vi "CRYGet Resolution_Steps of Curves.vi"(11 "Curve In":T1={"Name"="", "Curve"=[], "X data"=1, "Y data"=1, "Z data"=1, "X axis"=0, "Y axis"=1, "Z axis"=1, "X unit"="Hz", "Y unit"="", "Z unit"="deg.", "X dB ref"=1.0, "Y dB ref"=1.0, "Z dB ref"=1.0, "single val"=FALSE, "protected"=FALSE, "display X"=TRUE, "display Y"=TRUE, "display Z"=TRUE, "Test Info"="", "Step No."=0, "Plot Settings"={"Color"=0, "Interpolation"=0, "Point Style"=0, "Line Style"=0, "Point Color"=0, "Line Width"=0, "Bar Plot Style"=0, "Fill To"=0}, "AutoProtect"=FALSE} {"Z data" items=["dB", "Lin"]; "X data" items=["dB", "Lin"]; "Y data" items=["dB", "Lin"]; "Z dB ref" format="%.1f"; "Z axis" items=["Log", "Lin"]; "X dB ref" format="%.1f"; "X axis" items=["Log", "Lin"]; "Y axis" items=["Log", "Lin"]; "Y dB ref" format="%.1f"; "Curve"."z" format="%.2f"; "Curve"."y" format="%.2f"; "Curve"."x" format="%.2f"}) -> (1 "Steps Out":i32, 3 "Original Resolution Out":string)   [LabVIEW 2013]
uses:
  Typedef Control/CRYData Cluster.ctl
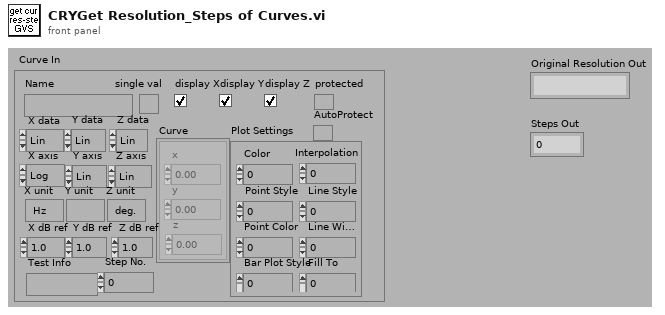
[diagram p1: front panel]
types:
  T1 = typedef "CRYData Cluster.ctl" = cluster{"Name":string, "Curve":cluster{"x":dbl, "y":dbl, "z":dbl}[], "X data":u16, "Y data":u16, "Z data":u16, "X axis":u16, "Y axis":u16, "Z axis":u16, "X unit":string, "Y unit":string, "Z unit":string, "X dB ref":dbl, "Y dB ref":dbl, "Z dB ref":dbl, "single val":bool, "protected":bool, "display X":bool, "display Y":bool, "display Z":bool, "Test Info":string, "Step No.":i32, "Plot Settings":cluster{"Color":u32, "Interpolation":u8, "Point Style":u8, "Line Style":u8, "Point Color":u32, "Line Width":u8, "Bar Plot Style":u8, "Fill To":i16}, "AutoProtect":bool}
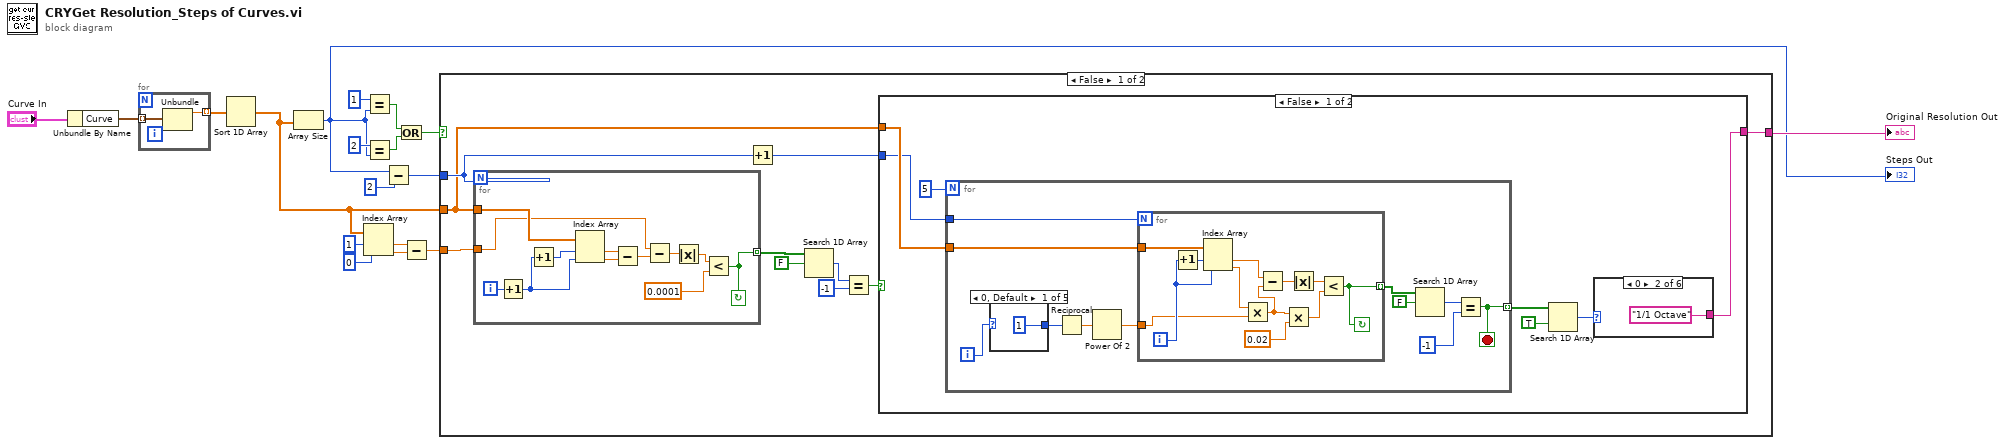
[diagram p0: block diagram]
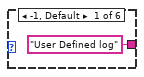
[diagram p2: hidden frame]
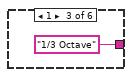
[diagram p3: hidden frame]
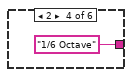
[diagram p4: hidden frame]
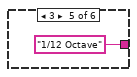
[diagram p5: hidden frame]
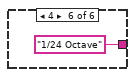
[diagram p6: hidden frame]
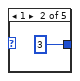
[diagram p7: hidden frame]
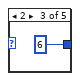
[diagram p8: hidden frame]
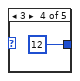
[diagram p9: hidden frame]
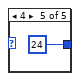
[diagram p10: hidden frame]
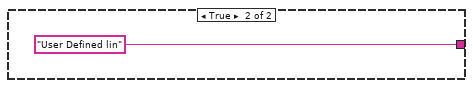
[diagram p11: hidden frame]
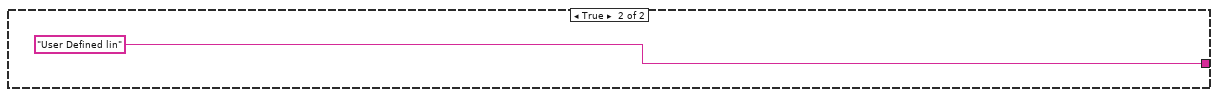
[diagram p12: hidden frame]
diagram:
  n1 = Unbundle By Name("Curve In") -> ("Curve"=w11:cluster{"x":dbl, "y":dbl, "z":dbl}[])
  n2 = for {
    tunnel: w11 -> [w20] mode=indexing
    tunnel: [w19] -> w2 mode=indexing
    n3 = Unbundle(w20) -> ("x"=w19:dbl)  [unwired: 2 out]
  }
  n4 = Sort 1D Array(array=w2) -> (sorted array=w1:dbl[])
  n5 = Array Size(array=w1) -> (size(s)=w4:i32)
  "Steps Out" <- w4
  n6 = Index Array(array=w1, index #1=1 ("index"), index #2=0 ("index")) -> (element #1=w9:dbl, element #2=w10:dbl)
  n7 = Equal?(x=1, y=w4) -> (x = y?=w15:bool)
  n8 = Equal?(x=2, y=w4) -> (x = y?=w14:bool)
  n9 = Subtract(x=w4, y=2) -> (x-y=w3:i32)
  n10 = Or(x=w15, y=w14) -> (x .or. y?=w13:bool)
  n11 = Subtract(x=w9, y=w10) -> (x-y=w6:dbl)
  n12 = case shown="False" w13 {
    tunnel: [w25 "User Defined lin"] -> w12
    tunnel: w3 -> [w23 _]
    tunnel: w1 -> [w22 _]
    tunnel: w6 -> [w24 _]
    frame False {
      n13 = for {
        N: w23 -> [_]
        tunnel: w22 -> [w84]
        tunnel: w24 -> [w78]
        tunnel: [w74] -> w30 mode=indexing
        i -> [w82]
        stop <- w74 continue-if-true
        n14 = Increment(x=w82) -> (x+1=w79:i32)
        n15 = Increment(x=w79) -> (x+1=w83:i32)
        n16 = Index Array(array=w84, index #1=w83, index #2=w79) -> (element #1=w81:dbl, element #2=w80:dbl)
        n17 = Subtract(x=w81, y=w80) -> (x-y=w75:dbl)
        n18 = Subtract(x=w78, y=w75) -> (x-y=w77:dbl)
        n19 = Absolute Value(x=w77) -> (abs(x)=w76:dbl)
        n20 = Less?(x=w76, y=0.0001) -> (x < y?=w74:bool)
      }
      n21 = Increment(x=w23) -> (x+1=w21:i32)
      n22 = Search 1D Array(1D array=w30, element=FALSE) -> (index of element=w28:i32)  [unwired: 1 in]
      n23 = Equal?(x=w28, y=-1) -> (x = y?=w26:bool)
      n24 = case shown="False" w26 {
        tunnel: [w36 "User Defined lin"] -> w25
        tunnel: w21 -> [w35 _]
        tunnel: w22 -> [w37 _]
        frame False {
          n25 = for {
            N: 5 -> [_]
            tunnel: w37 -> [w52]
            tunnel: w35 -> [w51]
            tunnel: [w44] -> w33 mode=indexing
            i -> [w45]
            stop <- w44 stop-if-true
            n26 = case shown="0, Default" w45 {
              tunnel: [1 3 6 12 24] -> w46
              frame 0, Default {
              }
              frame 1 {
              }
              frame 2 {
              }
              frame 3 {
              }
              frame 4 {
              }
            }
            n27 = Reciprocal(x=w46) -> (1/x=w54:dbl)
            n28 = Power Of 2(x=w54) -> (2^x=w53:dbl)
            n29 = for {
              N: w51 -> [_]
              tunnel: w53 -> [w63]
              tunnel: w52 -> [w66]
              tunnel: [w58] -> w50 mode=indexing
              i -> [w65]
              stop <- w58 continue-if-true
              n30 = Increment(x=w65) -> (x+1=w64:i32)
              n31 = Index Array(array=w66, index #1=w64, index #2=w65) -> (element #1=w61:dbl, element #2=w62:dbl)
              n32 = Multiply(x=w62, y=w63) -> (x*y=w57:dbl)
              n33 = Subtract(x=w61, y=w57) -> (x-y=w60:dbl)
              n34 = Multiply(x=w57, y=0.02) -> (x*y=w55:dbl)
              n35 = Absolute Value(x=w60) -> (abs(x)=w59:dbl)
              n36 = Less?(x=w59, y=w55) -> (x < y?=w58:bool)
            }
            n37 = Search 1D Array(1D array=w50, element=FALSE) -> (index of element=w48:i32)  [unwired: 1 in]
            n38 = Equal?(x=w48, y=-1) -> (x = y?=w44:bool)
          }
          n39 = Search 1D Array(1D array=w33, element=TRUE) -> (index of element=w31:i32)  [unwired: 1 in]
          n40 = case shown="0" w31 {
            tunnel: ["User Defined log" "1/1 Octave" "1/3 Octave" "1/6 Octave" "1/12 Octave" "1/24 Octave"] -> w36
            frame -1, Default {
            }
            frame 0 {
            }
            frame 1 {
            }
            frame 2 {
            }
            frame 3 {
            }
            frame 4 {
            }
          }
        }
        frame True {
        }
      }
    }
    frame True {
    }
  }
  "Original Resolution Out" <- w12
